vi "Find Device.vi"(5 "Address":u32, 6 "Baud Rate":u32=9600, 7 "Device Type":T1=enum."RS232", 8 "error in (no error)":errorcluster, 9 "Ports in Use":string[](array[string]), 10 "ID Response":string, 11 "ID String":string) -> (0 "error out":errorcluster, 1 "Device Found":bool, 2 "device ID":string, 3 "VISA resource name out":refnum<visa-resource-name>, 4 "read buffer":string)   [LabVIEW 2018, in "Utilities.lvlib"]
uses:
  Utilities.lvlib
  Find Device Protocols.ctl
  <vilib>/Instr/_visa.llb/VISA Find Search Mode.ctl
  <vilib>/Instr/_visa.llb/VISA Open Access Mode.ctl
  Hardware/Hardware Globals.vi
panel:
  out "read buffer clear":string
  # "V2.0"
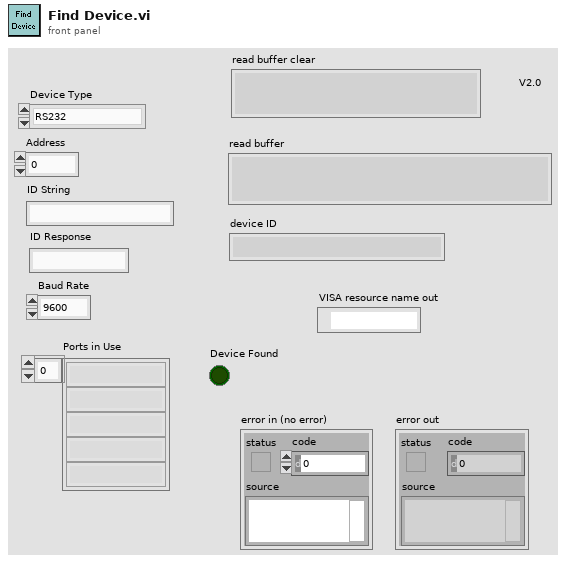
[diagram p1: front panel]
types:
  T1 = typedef "Find Device Protocols.ctl" = enum16{"Init", "RS232(no baud)", "RS232", "RS485", "USB", "GPIB", "Ethernet"}
  T2 = typedef "VISA Find Search Mode.ctl" = u32
  T3 = typedef "VISA Open Access Mode.ctl" = u32
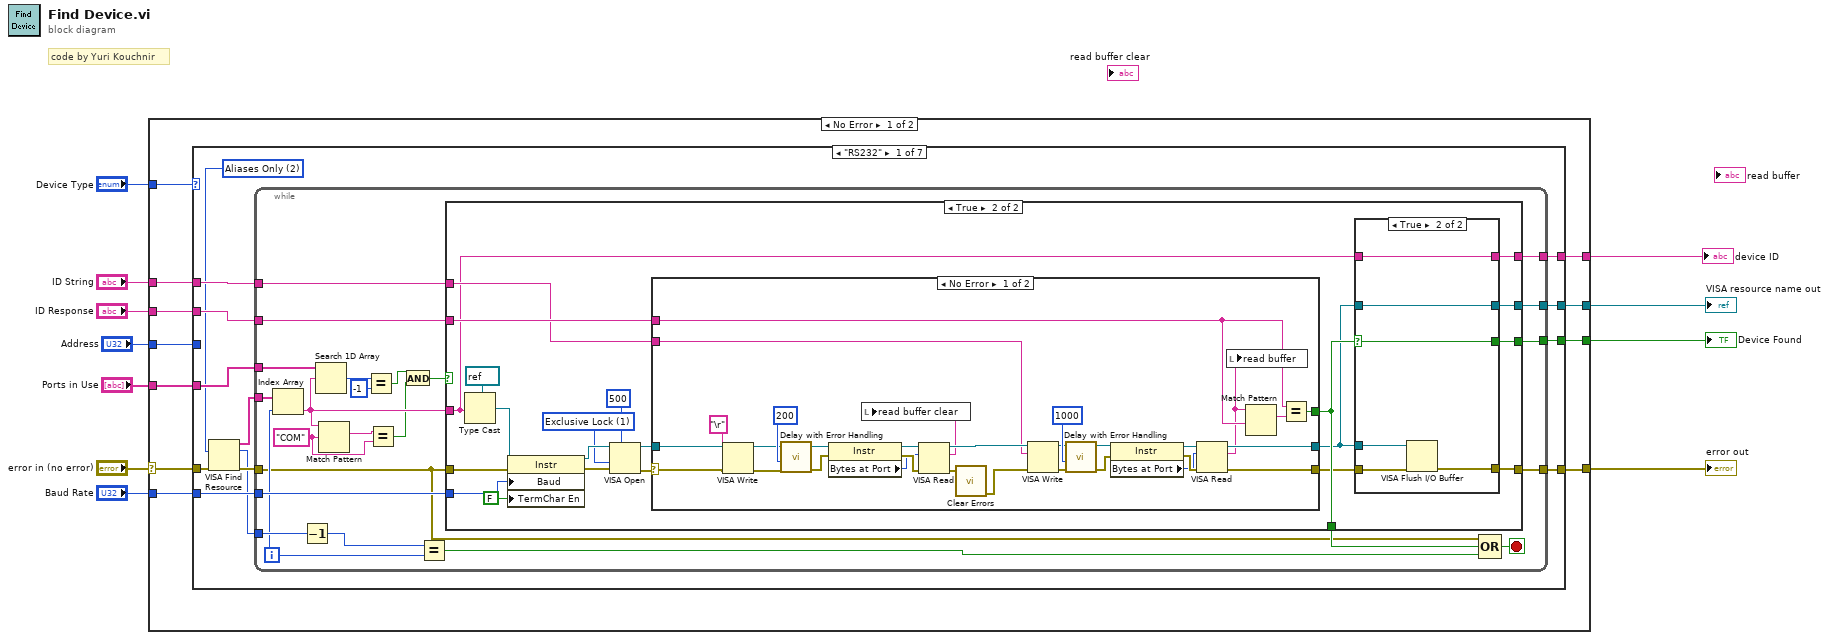
[diagram p0: block diagram]
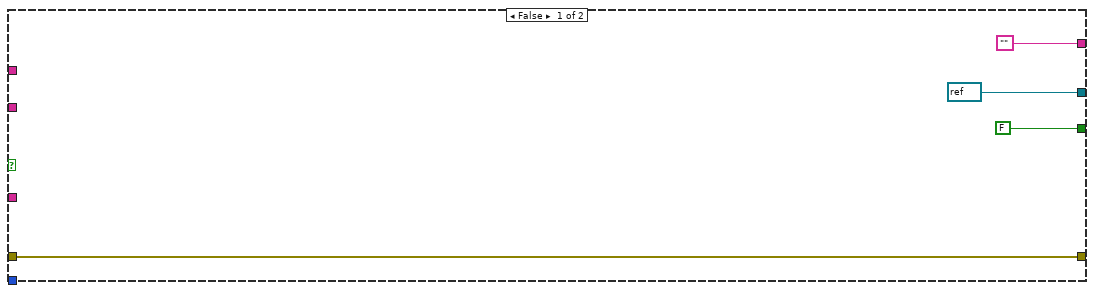
[diagram p2: hidden frame]
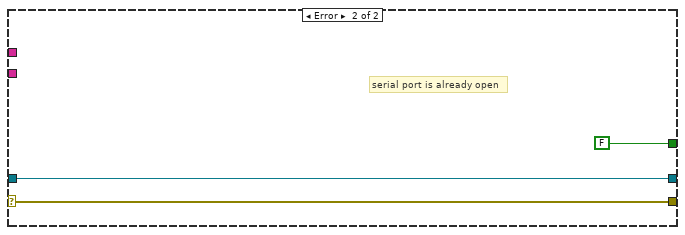
[diagram p3: hidden frame]
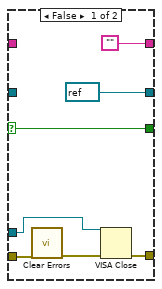
[diagram p4: hidden frame]
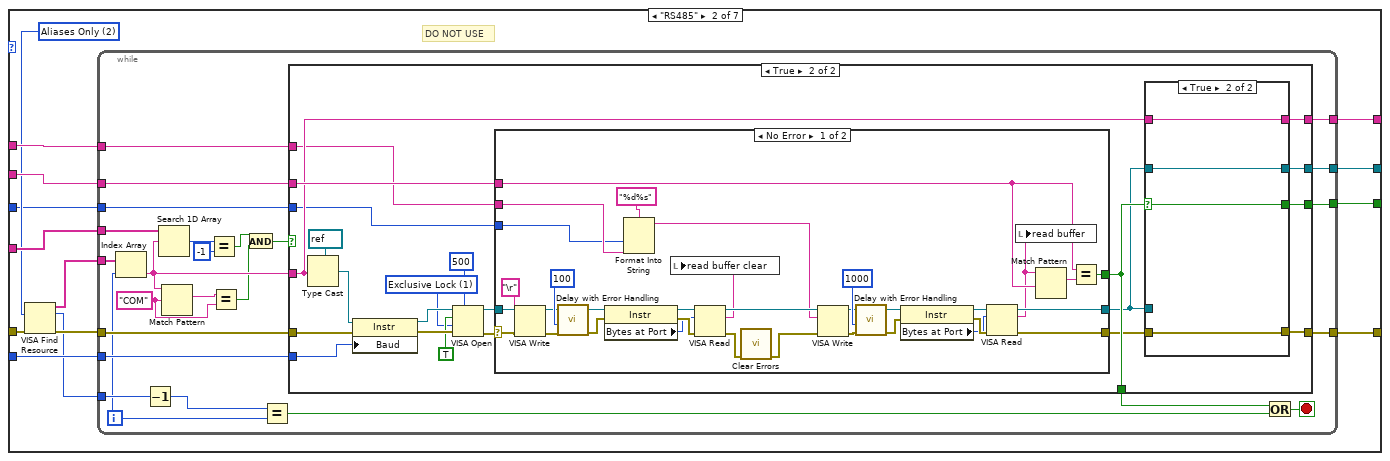
[diagram p5: hidden frame]
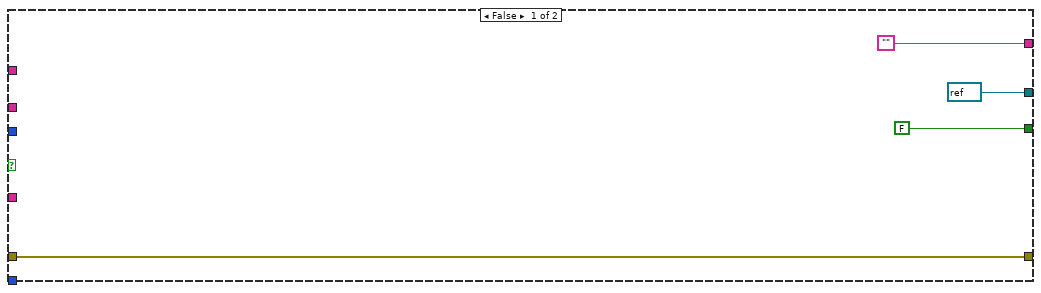
[diagram p6: hidden frame]
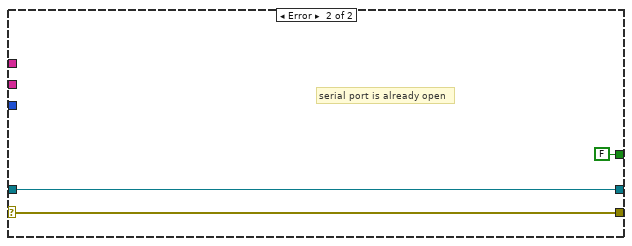
[diagram p7: hidden frame]
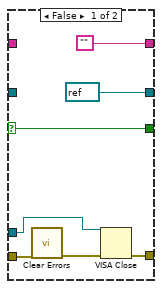
[diagram p8: hidden frame]
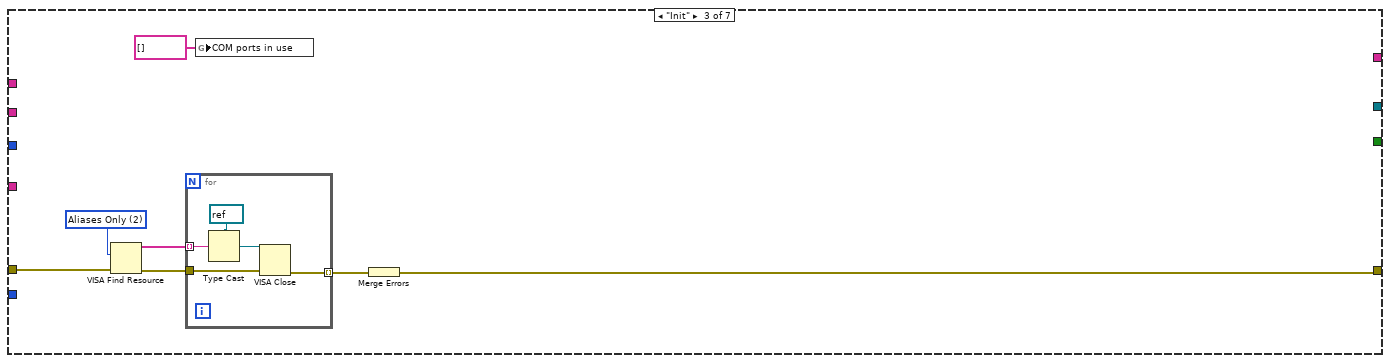
[diagram p9: hidden frame]
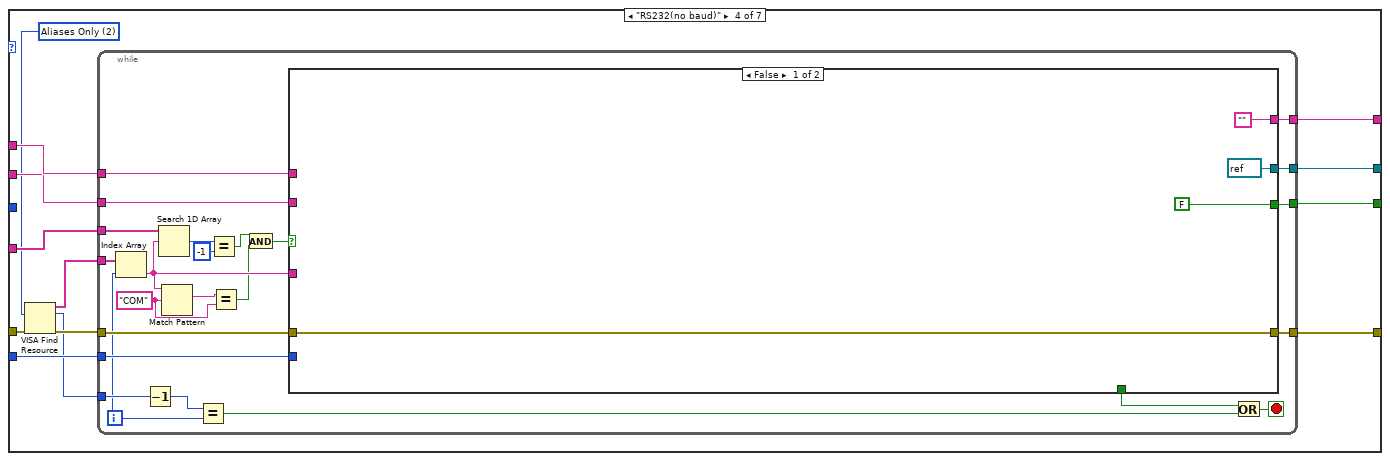
[diagram p10: hidden frame]
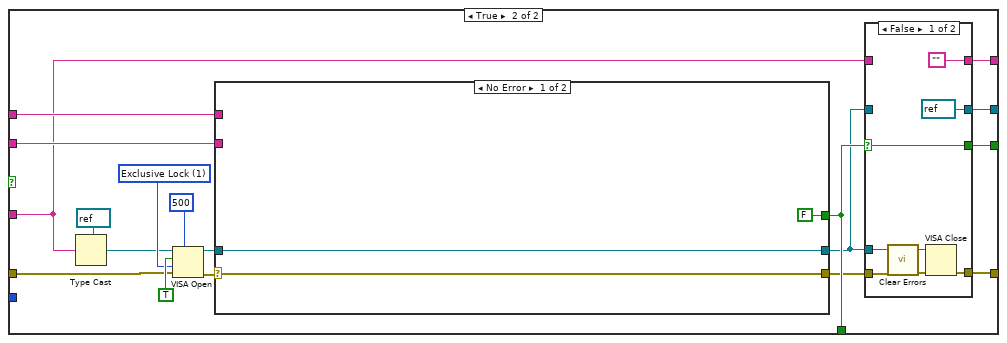
[diagram p11: hidden frame]
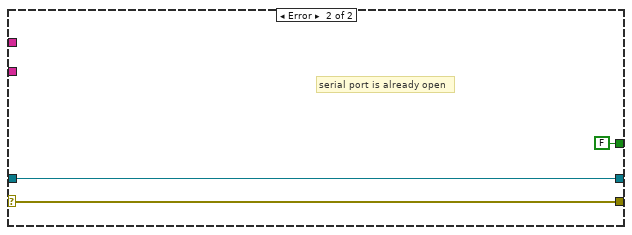
[diagram p12: hidden frame]
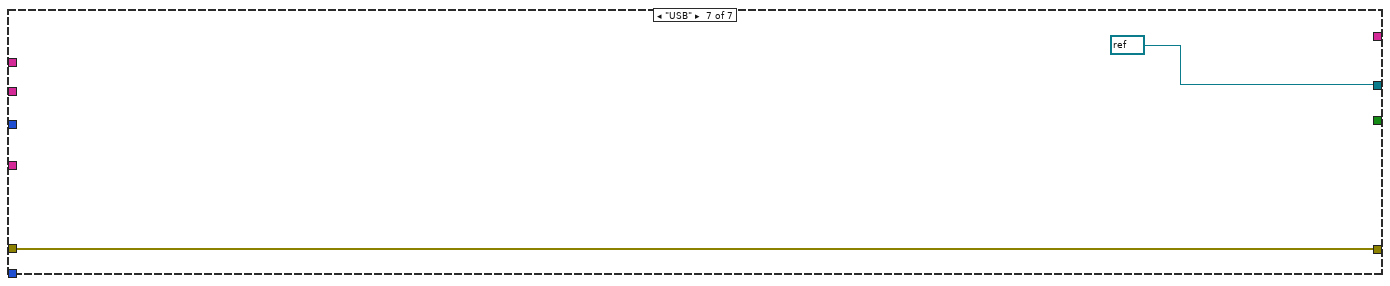
[diagram p16: hidden frame]
diagram:
  # "code by Yuri Kouchnir"
  n1 = case shown="No Error" "error in (no error)" {
    selector: "error in (no error)" -> [w21 _]
    tunnel: [w17 _] -> w11
    tunnel: "Device Type" -> [w22 _]
    tunnel: "ID String" -> [w20 _]
    tunnel: [w19 _] -> w4
    tunnel: [w18 _] -> w7
    tunnel: "Ports in Use" -> [w16 _]
    tunnel: "Baud Rate" -> [w15 _]
    tunnel: "ID Response" -> [w14 _]
    tunnel: "Address" -> [w13 _]
    tunnel: [w12 _] -> w1
    frame No Error {
      n2 = case shown="\"RS232\"" w22 {
        tunnel: w21 -> [w28 w135 w243 w256 w327 w328 w330]
        tunnel: w20 -> [w33 w140 _ w261 _ _ _]
        tunnel: [w30 w137 _ w258 _ _ refnum<visa-resource-name> refnum ("VISA resource name out")] -> w19
        tunnel: [w31 w138 _ w259 _ _ _] -> w18
        tunnel: [w29 w136 w239 w257 w327 w328 w330] -> w17
        tunnel: w16 -> [w35 w142 _ w263 _ _ _]
        tunnel: w15 -> [w34 w141 _ w262 _ _ _]
        tunnel: w14 -> [w32 w139 _ w260 _ _ _]
        tunnel: w13 -> [_ w130 _ _ _ _ _]
        tunnel: [w23 w129 _ w251 _ _ _] -> w12
        frame "RS232" {
          w24 = T2 2 items=["Canonical Names Only"=0, "Aliases Only"=2, "Include Matching Aliases"=3, "Include All Aliases"=4] ("Search Mode")
          n3 = VISA Find Resource(8:w28, 10:w24) -> (0:w27:errorcluster, 2:w26:u32, 3:w25:string[])  [unwired: 1 in]
          n4 = while {
            tunnel: w35 -> [w58]
            tunnel: w25 -> [w59]
            tunnel: w27 -> [w36]
            tunnel: w34 -> [w57]
            tunnel: w33 -> [w56]
            tunnel: w32 -> [w55]
            tunnel: w26 -> [w40]
            tunnel: [w50] -> w31
            tunnel: [w52] -> w30
            tunnel: [w49] -> w29
            tunnel: [w37] -> w23
            i -> [w39]
            stop <- w54 stop-if-true
            w44 = "COM" ("regular expression")
            n5 = Index Array(array=w59, index=w39) -> (element=w46:string)
            n6 = Decrement(x=w40) -> (x-1=w38:u32)
            n7 = Search 1D Array(1D array=w58, element=w46) -> (index of element=w48:i32)  [unwired: 1 in]
            n8 = Match Pattern(string=w46, regular expression=w44) -> (match substring=w45:string)  [unwired: 1 in, 3 out]
            n9 = Equal?(x=w48, y=-1) -> (x = y?=w43:bool)
            n10 = Equal?(x=w45, y=w44) -> (x = y?=w41:bool)
            n11 = And(x=w43, y=w41) -> (x .and. y?=w42:bool)
            n12 = Equal?(x=w38, y=w39) -> (x = y?=w53:bool)
            n13 = case shown="True" w42 {
              tunnel: w36 -> [w62 w77]
              tunnel: w46 -> [_ w66]
              tunnel: w57 -> [_ w79]
              tunnel: w56 -> [_ w72]
              tunnel: w55 -> [_ w81]
              tunnel: [refnum<visa-resource-name> refnum ("VISA resource name out") w84] -> w52
              tunnel: [_ w83] -> w51
              tunnel: [FALSE w82] -> w50
              tunnel: [w62 w68] -> w49
              tunnel: ["" w65] -> w37
              frame False {
              }
              frame True {
                w74 = T3 1 items=["VISA Defaults"=0, "Exclusive Lock"=1, "Load Configured Settings"=4] ("Access Mode")
                n14 = Type Cast(type=refnum<visa-resource-name> refnum ("VISA resource name"), x=w66) -> (*(type *) &x=w78:refnum<visa-resource-name>)
                n15 = property class="Instr"(reference=w78, error in=w77, "Baud"=w79, "TermChar En"=FALSE ("Message Based Settings:Termination Character Enable")) -> (reference out=w75:refnum<visa-resource-name>, error out=w76:errorcluster)
                n16 = VISA Open(timeout (0)=u32 500 ("VISA Open timeout (0)"), access mode=w74, error in (no error)=w76, VISA resource name=w75) -> (VISA resource name=w73:refnum<visa-resource-name>, error out=w71:errorcluster)  [unwired: 1 in]
                n17 = case shown="No Error" w71 {
                  selector: w71 -> [w96 w113]
                  tunnel: [w111 FALSE] -> w83
                  tunnel: [w110 w113] -> w69
                  tunnel: w81 -> [w109 _]
                  tunnel: [w108 w115] -> w67
                  tunnel: w73 -> [w97 w115]
                  tunnel: w72 -> [w103 _]
                  frame No Error {
                    n18 = VISA Write(VISA resource name=w97, write buffer="\r", error in (no error)=w96) -> (VISA resource name out=w87:refnum<visa-resource-name>, error out=w89:errorcluster)  [unwired: 1 out]
                    n19 = call "Delay with Error Handling.vi"("error in (no error)"=w89, "Delay (ms)"=u32 200 ("timeout (10sec)")) -> ("error out"=w88:errorcluster)  [unwired: 9 in]
                    n20 = property class="Instr"(reference=w87, error in=w88) -> (reference out=w93:refnum<visa-resource-name>, error out=w92:errorcluster, "Bytes at Port"=w91:u32)
                    n21 = VISA Read(VISA resource name=w93, byte count=w91, error in (no error)=w92) -> (VISA resource name out=w107:refnum<visa-resource-name>, read buffer=w86:string, error out=w94:errorcluster)  [unwired: 1 out]
                    n22 = local write "read buffer clear"(w86) -> ()
                    n23 = call <vilib>:"Clear Errors.vi"("error in (no error)"=w94) -> ("error out"=w106:errorcluster)  [unwired: 5 in, 1 out]
                    n24 = VISA Write(VISA resource name=w107, write buffer=w103, error in (no error)=w106) -> (VISA resource name out=w101:refnum<visa-resource-name>, error out=w105:errorcluster)  [unwired: 1 out]
                    n25 = call "Delay with Error Handling.vi"("error in (no error)"=w105, "Delay (ms)"=u32 1000 ("timeout (10sec)")) -> ("error out"=w100:errorcluster)  [unwired: 9 in]
                    n26 = property class="Instr"(reference=w101, error in=w100) -> (reference out=w102:refnum<visa-resource-name>, error out=w99:errorcluster, "Bytes at Port"=w98:u32)
                    n27 = VISA Read(VISA resource name=w102, byte count=w98, error in (no error)=w99) -> (VISA resource name out=w108:refnum<visa-resource-name>, read buffer=w95:string, error out=w110:errorcluster)  [unwired: 1 out]
                    n28 = local write "read buffer"(w95) -> ()
                    n29 = Match Pattern(string=w95, regular expression=w109) -> (match substring=w112:string)  [unwired: 1 in, 3 out]
                    n30 = Equal?(x=w109, y=w112) -> (x = y?=w111:bool)
                  }
                  frame Error {
                    # "serial port is already open"
                  }
                }
                n31 = case shown="True" w83 {
                  selector: w83 -> [w122 w128]
                  tunnel: w67 -> [_ w127]
                  tunnel: [refnum<visa-resource-name> refnum ("VISA resource name out") w127] -> w84
                  tunnel: [w122 w128] -> w82
                  tunnel: w69 -> [w119 w125]
                  tunnel: [w118 w124] -> w68
                  tunnel: w67 -> [w117 w123]
                  tunnel: w66 -> [_ w126]
                  tunnel: ["" w126] -> w65
                  frame False {
                    n32 = call <vilib>:"Clear Errors.vi"("error in (no error)"=w119) -> ("error out"=w120:errorcluster)  [unwired: 5 in, 1 out]
                    n33 = VISA Close(VISA resource name=w117, error in (no error)=w120) -> (error out=w118:errorcluster)
                  }
                  frame True {
                    n34 = VISA Flush I/O Buffer(VISA resource name=w123, error in (no error)=w125) -> (error out=w124:errorcluster)  [unwired: 1 in, 1 out]
                  }
                }
              }
            }
            n35 = Compound Arithmetic op=OR(w36, w51, w53) -> (w54:bool)
          }
        }
        frame "RS485" {
          w131 = T2 2 items=["Canonical Names Only"=0, "Aliases Only"=2, "Include Matching Aliases"=3, "Include All Aliases"=4] ("Search Mode")
          # "DO NOT USE"
          n36 = VISA Find Resource(8:w135, 10:w131) -> (0:w134:errorcluster, 2:w133:u32, 3:w132:string[])  [unwired: 1 in]
          n37 = while {
            tunnel: w142 -> [w166]
            tunnel: w132 -> [w167]
            tunnel: w134 -> [w165]
            tunnel: w141 -> [w164]
            tunnel: w140 -> [w163]
            tunnel: w139 -> [w162]
            tunnel: w133 -> [w146]
            tunnel: [w156] -> w138
            tunnel: [w159] -> w137
            tunnel: [w158] -> w129
            tunnel: [w155] -> w136
            tunnel: w130 -> [w143]
            i -> [w145]
            stop <- w161 stop-if-true
            w150 = "COM" ("regular expression")
            n38 = Index Array(array=w167, index=w145) -> (element=w152:string)
            n39 = Decrement(x=w146) -> (x-1=w144:u32)
            n40 = Search 1D Array(1D array=w166, element=w152) -> (index of element=w154:i32)  [unwired: 1 in]
            n41 = Match Pattern(string=w152, regular expression=w150) -> (match substring=w151:string)  [unwired: 1 in, 3 out]
            n42 = Equal?(x=w154, y=-1) -> (x = y?=w149:bool)
            n43 = Equal?(x=w151, y=w150) -> (x = y?=w147:bool)
            n44 = And(x=w149, y=w147) -> (x .and. y?=w148:bool)
            n45 = Equal?(x=w144, y=w145) -> (x = y?=w160:bool)
            n46 = case shown="True" w148 {
              tunnel: w165 -> [w169 w184]
              tunnel: w152 -> [_ w187]
              tunnel: w164 -> [_ w186]
              tunnel: w163 -> [_ w178]
              tunnel: w162 -> [_ w189]
              tunnel: [refnum<visa-resource-name> refnum ("VISA resource name out") w193] -> w159
              tunnel: ["" w192] -> w158
              tunnel: [_ w191] -> w157
              tunnel: [FALSE w190] -> w156
              tunnel: [w169 w174] -> w155
              tunnel: w143 -> [_ w172]
              frame False {
              }
              frame True {
                w180 = T3 1 items=["VISA Defaults"=0, "Exclusive Lock"=1, "Load Configured Settings"=4] ("Access Mode")
                n47 = Type Cast(type=refnum<visa-resource-name> refnum ("VISA resource name"), x=w187) -> (*(type *) &x=w185:refnum<visa-resource-name>)
                n48 = property class="Instr"(reference=w185, error in=w184, "Baud"=w186) -> (reference out=w182:refnum<visa-resource-name>, error out=w183:errorcluster)
                n49 = VISA Open(timeout (0)=u32 500 ("VISA Open timeout (0)"), duplicate session (F)=TRUE, access mode=w180, error in (no error)=w183, VISA resource name=w182) -> (VISA resource name=w179:refnum<visa-resource-name>, error out=w177:errorcluster)
                n50 = case shown="No Error" w177 {
                  selector: w177 -> [w208 w225]
                  tunnel: [w223 FALSE] -> w191
                  tunnel: [w222 w225] -> w175
                  tunnel: w189 -> [w221 _]
                  tunnel: [w220 w227] -> w173
                  tunnel: w179 -> [w209 w227]
                  tunnel: w178 -> [w195 _]
                  tunnel: w172 -> [w194 _]
                  frame No Error {
                    n51 = VISA Write(VISA resource name=w209, write buffer="\r", error in (no error)=w208) -> (VISA resource name out=w200:refnum<visa-resource-name>, error out=w202:errorcluster)  [unwired: 1 out]
                    n52 = call "Delay with Error Handling.vi"("error in (no error)"=w202, "Delay (ms)"=u32 100 ("timeout (10sec)")) -> ("error out"=w201:errorcluster)  [unwired: 9 in]
                    n53 = property class="Instr"(reference=w200, error in=w201) -> (reference out=w206:refnum<visa-resource-name>, error out=w205:errorcluster, "Bytes at Port"=w204:u32)
                    n54 = Format Into String(format string="%d%s", w194, w195) -> (resulting string=w197:string)  [unwired: 2 in, 1 out]
                    n55 = VISA Read(VISA resource name=w206, byte count=w204, error in (no error)=w205) -> (VISA resource name out=w219:refnum<visa-resource-name>, read buffer=w199:string, error out=w218:errorcluster)  [unwired: 1 out]
                    n56 = local write "read buffer clear"(w199) -> ()
                    n57 = call <vilib>:"Clear Errors.vi"("error in (no error)"=w218) -> ("error out"=w217:errorcluster)  [unwired: 5 in, 1 out]
                    n58 = VISA Write(VISA resource name=w219, write buffer=w197, error in (no error)=w217) -> (VISA resource name out=w213:refnum<visa-resource-name>, error out=w216:errorcluster)  [unwired: 1 out]
                    n59 = call "Delay with Error Handling.vi"("error in (no error)"=w216, "Delay (ms)"=u32 1000 ("timeout (10sec)")) -> ("error out"=w212:errorcluster)  [unwired: 9 in]
                    n60 = property class="Instr"(reference=w213, error in=w212) -> (reference out=w214:refnum<visa-resource-name>, error out=w211:errorcluster, "Bytes at Port"=w210:u32)
                    n61 = VISA Read(VISA resource name=w214, byte count=w210, error in (no error)=w211) -> (VISA resource name out=w220:refnum<visa-resource-name>, read buffer=w198:string, error out=w222:errorcluster)  [unwired: 1 out]
                    n62 = local write "read buffer"(w198) -> ()
                    n63 = Match Pattern(string=w198, regular expression=w221) -> (match substring=w224:string)  [unwired: 1 in, 3 out]
                    n64 = Equal?(x=w221, y=w224) -> (x = y?=w223:bool)
                  }
                  frame Error {
                    # "serial port is already open"
                  }
                }
                n65 = case shown="True" w191 {
                  selector: w191 -> [w233 w238]
                  tunnel: w187 -> [_ w235]
                  tunnel: w173 -> [_ w237]
                  tunnel: [refnum<visa-resource-name> refnum ("VISA resource name out") w237] -> w193
                  tunnel: ["" w235] -> w192
                  tunnel: [w233 w238] -> w190
                  tunnel: w175 -> [w230 w236]
                  tunnel: [w229 w236] -> w174
                  tunnel: w173 -> [w228 _]
                  frame False {
                    n66 = call <vilib>:"Clear Errors.vi"("error in (no error)"=w230) -> ("error out"=w231:errorcluster)  [unwired: 5 in, 1 out]
                    n67 = VISA Close(VISA resource name=w228, error in (no error)=w231) -> (error out=w229:errorcluster)
                  }
                  frame True {
                  }
                }
              }
            }
            n68 = Or(x=w157, y=w160) -> (x .or. y?=w161:bool)
          }
        }
        frame "Init" {
          w244 = T2 2 items=["Canonical Names Only"=0, "Aliases Only"=2, "Include Matching Aliases"=3, "Include All Aliases"=4] ("Search Mode")
          n69 = VISA Find Resource(8:w243, 10:w244) -> (0:w241:errorcluster, 3:w242:string[])  [unwired: 1 in, 1 out]
          n70 = for {
            tunnel: w242 -> [w250] mode=indexing
            tunnel: w241 -> [w248]
            tunnel: [w246] -> w240 mode=indexing
            n71 = Type Cast(type=refnum<visa-resource-name> refnum ("VISA resource name"), x=w250) -> (*(type *) &x=w247:refnum<visa-resource-name>)
            n72 = VISA Close(VISA resource name=w247, error in (no error)=w248) -> (error out=w246:errorcluster)
          }
          n73 = global write "Hardware Globals.vi" "COM ports in use"(string[] [] ("COM ports in use")) -> ()
          n74 = Merge Errors(w240) -> (w239:errorcluster)
        }
        frame "RS232(no baud)" {
          w252 = T2 2 items=["Canonical Names Only"=0, "Aliases Only"=2, "Include Matching Aliases"=3, "Include All Aliases"=4] ("Search Mode")
          n75 = VISA Find Resource(8:w256, 10:w252) -> (0:w255:errorcluster, 2:w254:u32, 3:w253:string[])  [unwired: 1 in]
          n76 = while {
            tunnel: w263 -> [w286]
            tunnel: w253 -> [w287]
            tunnel: w255 -> [w285]
            tunnel: w262 -> [w284]
            tunnel: w261 -> [w283]
            tunnel: w260 -> [w282]
            tunnel: w254 -> [w267]
            tunnel: [w277] -> w259
            tunnel: [w279] -> w258
            tunnel: [w276] -> w257
            tunnel: [w264] -> w251
            i -> [w266]
            stop <- w281 stop-if-true
            w271 = "COM" ("regular expression")
            n77 = Index Array(array=w287, index=w266) -> (element=w273:string)
            n78 = Decrement(x=w267) -> (x-1=w265:u32)
            n79 = Search 1D Array(1D array=w286, element=w273) -> (index of element=w275:i32)  [unwired: 1 in]
            n80 = Match Pattern(string=w273, regular expression=w271) -> (match substring=w272:string)  [unwired: 1 in, 3 out]
            n81 = Equal?(x=w265, y=w266) -> (x = y?=w280:bool)
            n82 = Equal?(x=w275, y=-1) -> (x = y?=w270:bool)
            n83 = Equal?(x=w272, y=w271) -> (x = y?=w268:bool)
            n84 = And(x=w270, y=w268) -> (x .and. y?=w269:bool)
            n85 = case shown="False" w269 {
              tunnel: w285 -> [w290 w295]
              tunnel: w273 -> [_ w292]
              tunnel: w284 -> [_ _]
              tunnel: w283 -> [_ w301]
              tunnel: w282 -> [_ w306]
              tunnel: [refnum<visa-resource-name> refnum ("VISA resource name out") w309] -> w279
              tunnel: [_ w308] -> w278
              tunnel: [FALSE w307] -> w277
              tunnel: [w290 w297] -> w276
              tunnel: ["" w293] -> w264
              frame False {
              }
              frame True {
                w303 = T3 1 items=["VISA Defaults"=0, "Exclusive Lock"=1, "Load Configured Settings"=4] ("Access Mode")
                n86 = Type Cast(type=refnum<visa-resource-name> refnum ("VISA resource name"), x=w292) -> (*(type *) &x=w294:refnum<visa-resource-name>)
                n87 = VISA Open(timeout (0)=u32 500 ("VISA Open timeout (0)"), duplicate session (F)=TRUE, access mode=w303, error in (no error)=w295, VISA resource name=w294) -> (VISA resource name=w302:refnum<visa-resource-name>, error out=w300:errorcluster)
                n88 = case shown="No Error" w300 {
                  selector: w300 -> [w312 w313]
                  tunnel: [FALSE FALSE] -> w308
                  tunnel: [w312 w313] -> w298
                  tunnel: w306 -> [_ _]
                  tunnel: [w311 w315] -> w296
                  tunnel: w302 -> [w311 w315]
                  tunnel: w301 -> [_ _]
                  frame No Error {
                  }
                  frame Error {
                    # "serial port is already open"
                  }
                }
                n89 = case shown="False" w308 {
                  selector: w308 -> [w322 w326]
                  tunnel: w296 -> [_ w325]
                  tunnel: [refnum<visa-resource-name> refnum ("VISA resource name out") w325] -> w309
                  tunnel: [w322 w326] -> w307
                  tunnel: w298 -> [w319 w324]
                  tunnel: [w318 w324] -> w297
                  tunnel: w296 -> [w317 _]
                  tunnel: ["" w323] -> w293
                  tunnel: w292 -> [_ w323]
                  frame False {
                    n90 = call <vilib>:"Clear Errors.vi"("error in (no error)"=w319) -> ("error out"=w320:errorcluster)  [unwired: 5 in, 1 out]
                    n91 = VISA Close(VISA resource name=w317, error in (no error)=w320) -> (error out=w318:errorcluster)
                  }
                  frame True {
                  }
                }
              }
            }
            n92 = Or(x=w278, y=w280) -> (x .or. y?=w281:bool)
          }
        }
        frame "GPIB" {
          # "not done yet"
        }
        frame "Ethernet" {
          # "not done yet"
        }
        frame "USB" {
        }
      }
    }
    frame Error {
    }
  }
  "error out" <- w11
  "Device Found" <- w7
  "VISA resource name out" <- w4
  "device ID" <- w1
